vi "Bin Winch tension measurement interface.vi"() -> (3 "Winch is loose":bool)   [LabVIEW 2014]
panel:
  out "String Pot Value":dbl
  in  "String Pot tension threshold":dbl=0.113
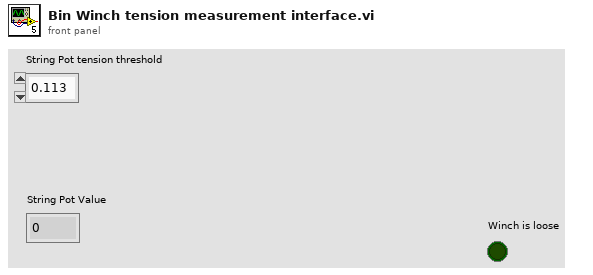
[diagram p1: front panel]
types:
  T1 = typedef "WPI_PotentiometerDevRef.ctl" = cluster{"DevStatus":errorcluster, "Controller":T2, "Analog Channel":T3, "Invert Output":bool}
  T2 = typedef "FPGA_TypedefAnalogModule.ctl" = enum16{"Controller 1"}
  T3 = typedef "FPGA_AIChannel.ctl" = enum8{"AI 0", "AI 1", "AI 2", "AI 3", "AI MXP 0", "AI MXP 1", "AI MXP 2", "AI MXP 3", "Invalid"}
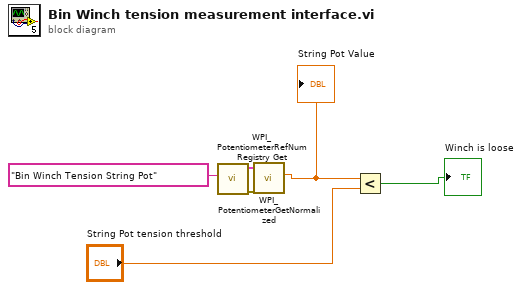
[diagram p0: block diagram]
diagram:
  n1 = call <vilib>:"WPI_PotentiometerRefNum Registry Get.vi"("refnum name"="Bin Winch Tension String Pot") -> ("error out"=w6:errorcluster, "PotDevRef"=w5:T1)  [unwired: 9 in]
  n2 = call <vilib>:"WPI_PotentiometerGetNormalized.vi"("error in"=w6, "PotDevRef"=w5) -> ("Normalized Value"=w3:dbl)  [unwired: 7 in, 2 out]
  "String Pot Value" <- w3
  n3 = Less?(x=w3, y="String Pot tension threshold") -> (x < y?=→"Winch is loose":bool)
